vi "Feeder Launcher.vi"(9 "Sub Panel":refnum<vi>, 10 "Feeder ID":enum16{"Main Feeder", "Secondary Feeder"}(ring), 11 "Panel Actor In":refnum<class "Main.lvclass">) -> (2 "Nested Actor's Enqueuer":refnum<class "Message Enqueuer.lvclass">, 3 "Panel Actor Out":refnum<class "Main.lvclass">)   [LabVIEW 2018, in "Feeder Actor.lvlib" / "Feeder.lvclass"]
uses:
  Feeder.lvclass
  ADM/ADM/Main.lvclass
  C:/Program Files/National Instruments/LabVIEW 2018/vi.lib/MGI/Panel Manager/Panel Actor/Panel Actor/Panel Actor.lvclass
  <vilib>/ActorFramework/Message Enqueuer/Message Enqueuer.lvclass
  Feeder.lvclass/Feeder.ctl
  <vilib>/MGI/Panel Manager/Panel/Panel/Subpanel/Subpanel.lvclass
  C:/Program Files/National Instruments/LabVIEW 2018/vi.lib/MGI/Panel Manager/Panel/Panel/Panel.lvclass
  <vilib>/MGI/Panel Manager/Panel/Panel/Subpanel/Subpanel.vi
  <vilib>/MGI/Panel Manager/Panel/Panel.lvlib
  <vilib>/MGI/Panel Manager/Panel Actor/Panel Actor/Panel Actor.lvclass
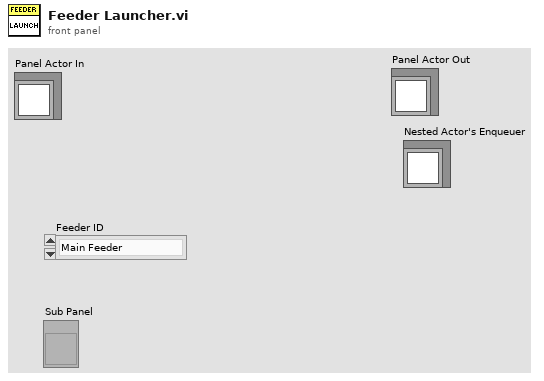
[diagram p1: front panel]
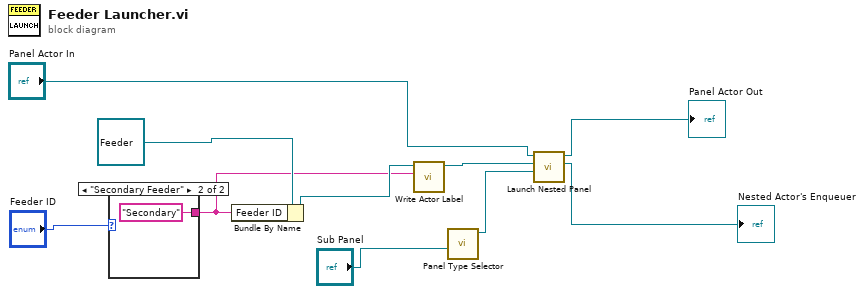
[diagram p0: block diagram]
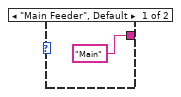
[diagram p2: hidden frame]
diagram:
  n1 = case shown="\"Secondary Feeder\"" "Feeder ID" {
    tunnel: ["Main" "Secondary"] -> w1
    frame "Main Feeder", Default {
    }
    frame "Secondary Feeder" {
    }
  }
  n2 = Bundle By Name(cluster=refnum<class "Feeder.lvclass"> refnum ("Feeder Actor.lvlib:Feeder.lvclass"), "Feeder ID"=w1) -> (w3:refnum<class "Feeder.lvclass">)
  n3 = call-dynamic "Write Actor Label.vi"("Actor Label"=w1, "Monitored Actor in"=w3) -> ("Monitored Actor out"=w2:refnum<class "Feeder.lvclass">)  [unwired: 8 in, 1 out]
  n4 = call-poly <vilib>:"Panel Type Selector.vi"("Sub Panel"="Sub Panel") -> ("Subpanel Out"=w6:refnum<class "Subpanel.lvclass">)  [unwired: 9 in, 1 out]
  n5 = call <vilib>:"Launch Nested Panel.vi"("Panel"=w6, "Nested Panel Actor"=w2, "Panel Actor in"="Panel Actor In") -> ("Nested Actor's Enqueuer"=→"Nested Actor's Enqueuer":refnum<class "Message Enqueuer.lvclass">, "Panel Actor out"=→"Panel Actor Out":refnum<class "Main.lvclass">)  [unwired: 5 in, 2 out]
